vi "Configure Marker Destination.vi"(6 "Alternate Amplitude (0: None)":u16(ring) items=["None", "Marker1", "Marker2", "Marker3", "Marker4"], 7 "Pulse (0: None)":u16(ring) items=["None", "Marker1", "Marker2", "Marker3", "Marker4"], 8 "error in (no error)":errorcluster, 9 "ALC Hold (0: None)":u16(ring) items=["None", "Marker1", "Marker2", "Marker3", "Marker4"], 10 "Modulation Format (1: Dual Modulation)":u16(ring)=1 items=["Dual Modulation"=1, "Dual ARB"=2, "Multitone"=3, "Two-tone"=6, "AWGN ARB"=8], 11 "VISA resource name":refnum<visa-resource-name>) -> (0 "error out":errorcluster, 3 "VISA resource name out":refnum<visa-resource-name>)   [LabVIEW 2014, in "Agilent PSG MXG Series.lvlib"]
doc: "Configures the marker pulse/RF function, ALC hold function and alternate amplitude for the specific modulation format.\n\n<B>Notes:</B>\n(1) This VI is valid only in E8267C, E8257D, E8267D, N5162A, N5182A, N5172B, N5182B.\n\n(2) For E8267C, this VI is valid only when the instrument installs <B>Option 002</B> (Internal baseband generator) or <B>Option 602</B> (Digital bus baseband generator).\n\n(3) For E8267D, this VI is valid only when the instrument installs <B>Option 601</B> or <B>Option 602</B> (Internal baseband generator).\n\n(4) For N5162A and N5182A, this VI is valid only when the instrument installs <B>Option 651</B> or <B>Option 652</B> or <B>Option 654</B> (Internal baseband generator), and <B>Option 432</B> (Phase noise impairment)."
uses:
  Agilent PSG MXG Series.lvlib
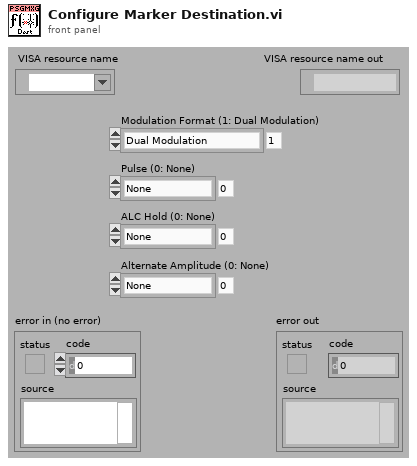
[diagram p1: front panel]
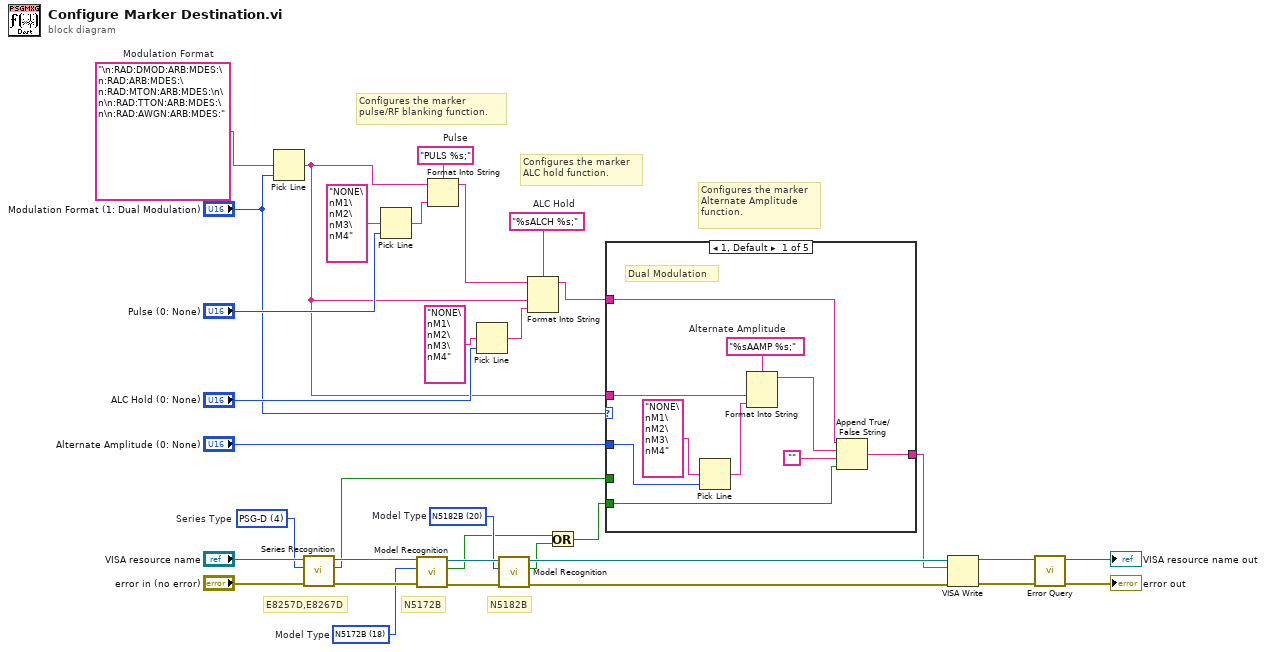
[diagram p0: block diagram]
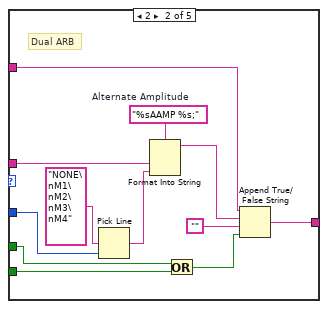
[diagram p2: hidden frame]
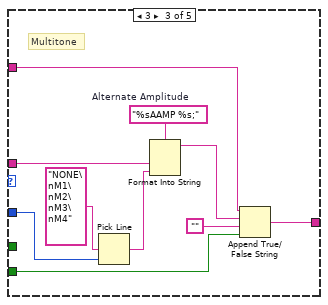
[diagram p3: hidden frame]
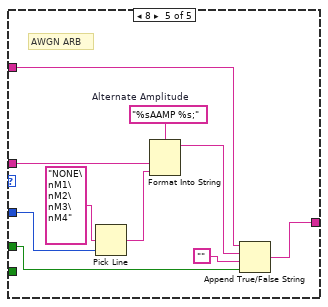
[diagram p5: hidden frame]
diagram:
  w10 = u16 20 items=["N5181A"=0, "N5182A"=1, "N5183A"=2, "N5161A"=3, "N5162A"=4, "E8241A"=5, "E8244A"=6, "E8251A"=7, "E8254A"=8, "E8247C"=10, "E8257C"=11, "E8267C"=12, "E8257D"=15, "E8267D"=16, "N5171B"=17, "N5172B"=18, "N5181B"=19, "N5182B"=20]  # Model Type
  w11 = u16 18 items=["N5181A"=0, "N5182A"=1, "N5183A"=2, "N5161A"=3, "N5162A"=4, "E8241A"=5, "E8244A"=6, "E8251A"=7, "E8254A"=8, "E8247C"=10, "E8257C"=11, "E8267C"=12, "E8257D"=15, "E8267D"=16, "N5171B"=17, "N5172B"=18, "N5181B"=19, "N5182B"=20]  # Model Type
  w18 = u16 4 items=["MXG-A", "PSG", "PSG-A", "PSG-C", "PSG-D", "MXG-B", "EXG"]  # Series Type
  w28 = "%sALCH %s;"  # ALC Hold
  w33 = "PULS %s;"  # Pulse
  w34 = "\n:RAD:DMOD:ARB:MDES:\n:RAD:ARB:MDES:\n:RAD:MTON:ARB:MDES:\n\n\n:RAD:TTON:ARB:MDES:\n\n:RAD:AWGN:ARB:MDES:"  # Modulation Format
  # "Configures the marker\nAlternate Amplitude\nfunction."
  # "N5182B"
  # "N5172B"
  # "E8257D,E8267D"
  # "Configures the marker\nALC hold function."
  # "Configures the marker\npulse/RF blanking function."
  n1 = Pick Line(multi-line string=w34, line index="Modulation Format (1: Dual Modulation)") -> (output string=w7:string)  [unwired: 1 out]
  n2 = call "Series Recognition.vi"("error in (no error)"="error in (no error)", "Series Type (0: MXG)"=w18, "VISA resource name"="VISA resource name") -> ("error out"=w16:errorcluster, "Is Series Correct"=w2:bool, "VISA resource name out"=w17:refnum<visa-resource-name>)  [unwired: 6 out]
  n3 = Pick Line(multi-line string="NONE\nM1\nM2\nM3\nM4", line index="Pulse (0: None)") -> (output string=w32:string)  [unwired: 1 out]
  n4 = call "Model Recognition.vi"("error in (no error)"=w16, "Model Type (0: N5181A)"=w11, "VISA resource name"=w17) -> ("error out"=w14:errorcluster, "Is Model Correct"=w4:bool, "VISA resource name out"=w15:refnum<visa-resource-name>)  [unwired: 6 out]
  n5 = Format Into String(format string=w33, initial string=w7, w32) -> (resulting string=w29:string)  [unwired: 1 in, 1 out]
  n6 = Pick Line(multi-line string="NONE\nM1\nM2\nM3\nM4", line index="ALC Hold (0: None)") -> (output string=w23:string)  [unwired: 1 out]
  n7 = call "Model Recognition.vi"("error in (no error)"=w14, "Model Type (0: N5181A)"=w10, "VISA resource name"=w15) -> ("error out"=w12:errorcluster, "Is Model Correct"=w5:bool, "VISA resource name out"=w13:refnum<visa-resource-name>)  [unwired: 6 out]
  n8 = Format Into String(format string=w28, initial string=w29, w7, w23) -> (resulting string=w8:string)  [unwired: 1 in, 1 out]
  n9 = Or(x=w4, y=w5) -> (x .or. y?=w3:bool)
  n10 = case shown="1, Default" "Modulation Format (1: Dual Modulation)" {
    tunnel: w8 -> [w39 w52 w62 w67 w73]
    tunnel: w7 -> [w41 w53 w63 _ w74]
    tunnel: "Alternate Amplitude (0: None)" -> [w35 w45 w57 _ w68]
    tunnel: w3 -> [w40 w46 w58 _ _]
    tunnel: w2 -> [_ w47 _ _ w69]
    tunnel: [w36 w49 w59 w67 w70] -> w1
    frame 1, Default {
      w44 = "%sAAMP %s;"  # Alternate Amplitude
      # "Dual Modulation"
      n11 = Pick Line(multi-line string="NONE\nM1\nM2\nM3\nM4", line index=w35) -> (output string=w43:string)  [unwired: 1 out]
      n12 = Format Into String(format string=w44, w41, w43) -> (resulting string=w38:string)  [unwired: 2 in, 1 out]
      n13 = Append True/False String(1:w40, 2:"", 3:w38, 4:w39) -> (0:w36:string)
    }
    frame 2 {
      w56 = "%sAAMP %s;"  # Alternate Amplitude
      # "Dual ARB"
      n14 = Pick Line(multi-line string="NONE\nM1\nM2\nM3\nM4", line index=w45) -> (output string=w55:string)  [unwired: 1 out]
      n15 = Format Into String(format string=w56, w53, w55) -> (resulting string=w51:string)  [unwired: 2 in, 1 out]
      n16 = Or(x=w47, y=w46) -> (x .or. y?=w48:bool)
      n17 = Append True/False String(1:w48, 2:"", 3:w51, 4:w52) -> (0:w49:string)
    }
    frame 3 {
      w66 = "%sAAMP %s;"  # Alternate Amplitude
      # "Multitone"
      n18 = Pick Line(multi-line string="NONE\nM1\nM2\nM3\nM4", line index=w57) -> (output string=w65:string)  [unwired: 1 out]
      n19 = Format Into String(format string=w66, w63, w65) -> (resulting string=w61:string)  [unwired: 2 in, 1 out]
      n20 = Append True/False String(1:w58, 2:"", 3:w61, 4:w62) -> (0:w59:string)
    }
    frame 6 {
      # "Two-tone"
    }
    frame 8 {
      w77 = "%sAAMP %s;"  # Alternate Amplitude
      # "AWGN ARB"
      n21 = Pick Line(multi-line string="NONE\nM1\nM2\nM3\nM4", line index=w68) -> (output string=w76:string)  [unwired: 1 out]
      n22 = Format Into String(format string=w77, w74, w76) -> (resulting string=w72:string)  [unwired: 2 in, 1 out]
      n23 = Append True/False String(1:w69, 2:"", 3:w72, 4:w73) -> (0:w70:string)
    }
  }
  n24 = VISA Write(VISA resource name=w13, write buffer=w1, error in (no error)=w12) -> (VISA resource name out=w25:refnum<visa-resource-name>, error out=w24:errorcluster)  [unwired: 1 out]
  n25 = call "Error Query.vi"("error in (no error)"=w24, "VISA resource name"=w25) -> ("error out"=→"error out":errorcluster, "VISA resource name out"=→"VISA resource name out":refnum<visa-resource-name>)  [unwired: 8 out]
